vi "Get Thread Configuration.vi"(8 "error in (no error)":errorcluster, 10 "index":i32, 11 "Plugin Configuration in":refnum<class "Plugin Configuration.lvclass">) -> (0 "error out":errorcluster, 2 "Thread Configuration":refnum<class "Thread Configuration.lvclass">, 3 "Plugin Configuration out":refnum<class "Plugin Configuration.lvclass">)   [LabVIEW 2020, in "DSF Core.lvlib" / "Plugin Configuration.lvclass"]
uses:
  Plugin Configuration.lvclass
  Thread/Thread Configuration.lvclass
  Plugin Configuration.lvclass/Plugin Configuration.ctl
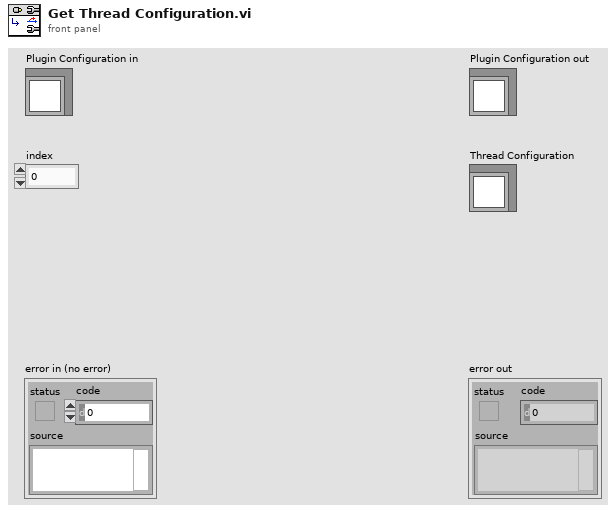
[diagram p1: front panel]
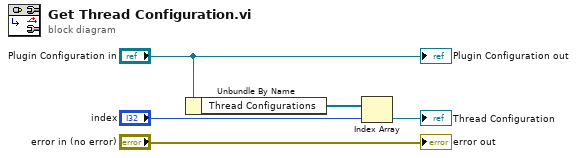
[diagram p0: block diagram]
diagram:
  n1 = Unbundle By Name("Plugin Configuration in") -> ("Thread Configurations"=w3:refnum<class "Thread Configuration.lvclass">[])
  n2 = Index Array(array=w3, index="index") -> (element=→"Thread Configuration":refnum<class "Thread Configuration.lvclass">)
  "error out" <- "error in (no error)"
  "Plugin Configuration out" <- "Plugin Configuration in"
